vi "csv to array (read from csv).vi"(6 "File Path in":path, 9 "select source":enum32{"user selectable", "constant"}(ring)) -> (1 "Array":string[](array[string]), 3 "all rows":string[][](array[string]))   [LabVIEW 2011]
uses:
  <vilib>/Utility/file.llb/Read From Spreadsheet File (string).vi
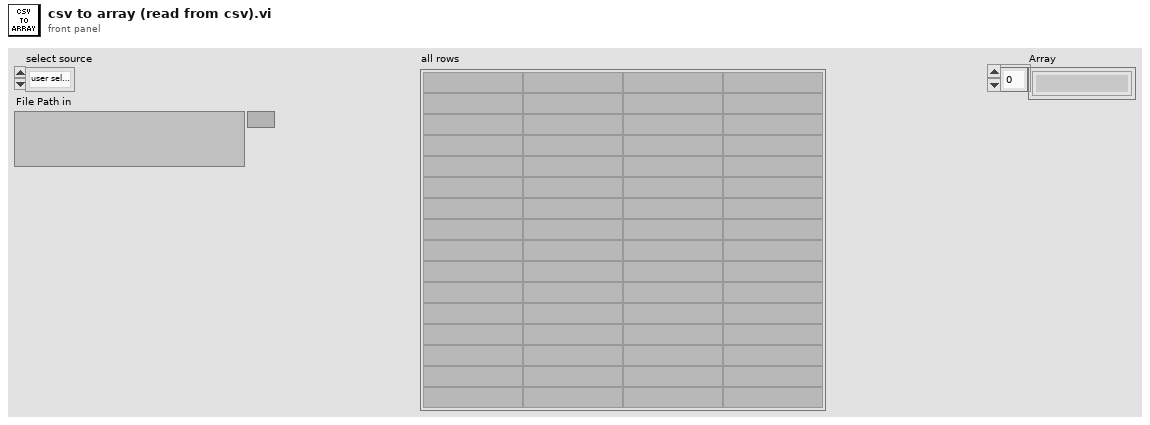
[diagram p1: front panel]
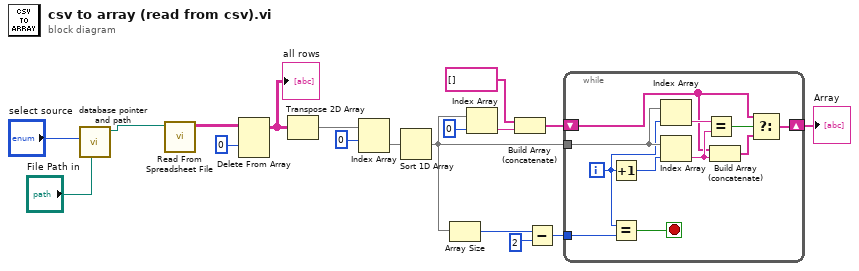
[diagram p0: block diagram]
diagram:
  n1 = call "database pointer and path.vi"("File Path in"="File Path in", "select source"="select source") -> ("appended path"=w3:path)  [unwired: 8 in, 1 out]
  n2 = call-poly <vilib>:"Read From Spreadsheet File.vi"("file path (dialog if empty)"=w3) -> ("all rows"=w15:string[][])  [unwired: 6 in, 4 out]
  n3 = Delete From Array(array=w15, index (row)=0) -> (array with subset deleted=w13:string[][])  [unwired: 2 in, 1 out]
  "all rows" <- w13
  n4 = Transpose 2D Array(2D array=w13) -> (transposed array=w17:string[][])
  n5 = Index Array(array=w17, index (row)=0) -> (element=w16:string[])  [unwired: 1 in]
  n6 = Sort 1D Array(array=w16) -> (sorted array=w6:string[])
  n7 = Array Size(array=w6) -> (size(s)=w8:i32)
  n8 = Index Array(array=w6, index=0) -> (element=w10:string)
  n9 = Build Array (concatenate)(string[] [], w10) -> (w12:string[])
  n10 = Subtract(x=w8, y=2) -> (x-y=w5:i32)
  n11 = while {
    tunnel: w6 -> [w28]
    shift-right: [w22] -> w4
    shift-left: w12 -> [w20]
    tunnel: w5 -> [w25]
    i -> [w24]
    stop <- w23 stop-if-true
    n12 = Increment(x=w24) -> (x+1=w29:i32)
    n13 = Equal?(x=w24, y=w25) -> (x = y?=w23:bool)
    n14 = Index Array(array=w28, index=w24) -> (element=w27:string)
    n15 = Index Array(array=w28, index=w29) -> (element=w21:string)
    n16 = Equal?(x=w27, y=w21) -> (x = y?=w26:bool)
    n17 = Build Array (concatenate)(w20, w21) -> (w19:string[])
    n18 = Select(t=w20, s=w26, f=w19) -> (s? t:f=w22:string[])
  }
  "Array" <- w4
